vi "test_easy_linear_interpl.vi"() -> ()   [LabVIEW 2009]
doc: "Copyright (C) 2009, Stepan A. Baranov\nweb: http://www.OCTLab.org/\nemail: stepan@baranov.su"
uses:
  OCTLib.dll
panel:
  out "RSM_STAT final 2D array":dbl[](array[numeric])
  out "error out":errorcluster
  out "data Graph":dynamicdata(graph)
  out "wavelengths Graph":dynamicdata(graph)
  out "LabView final 2D array":dbl[](array[numeric])
  out "initial 2D array":dbl[](array[numeric])
  in  "stop":bool
  in  "index (row)":i32=1
  in  "Y":i32=9
  in  "X":i32=800
  in  "End wavelength":dbl=890.0
  in  "Start wavelength":dbl=800.0
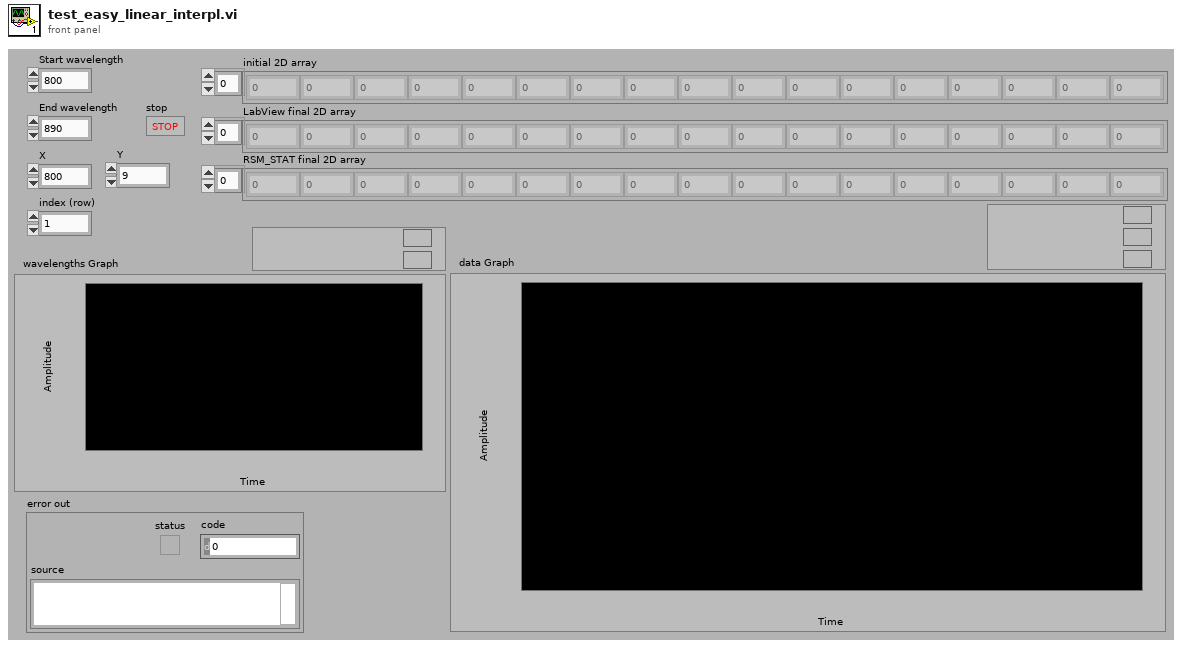
[diagram p1: front panel]
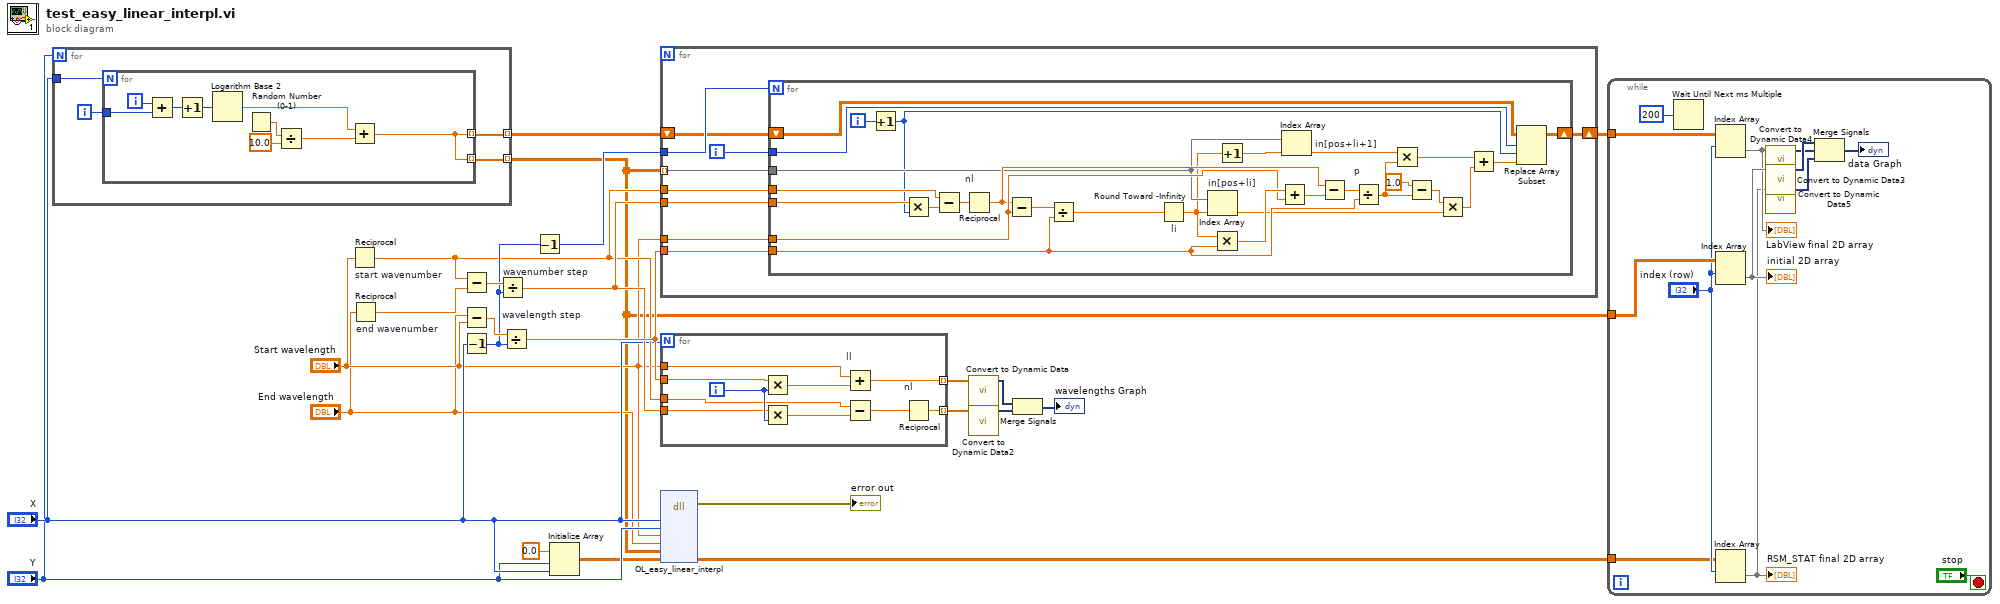
[diagram p0: block diagram]
diagram:
  n1 = for {
    N: "Y" -> [_]
    tunnel: [w28] -> w3 mode=indexing
    tunnel: "X" -> [w27]
    tunnel: [w26] -> w19 mode=indexing
    i -> [w25]
    n2 = for {
      N: w27 -> [_]
      tunnel: [w36] -> w28 mode=indexing
      tunnel: [w36] -> w26 mode=indexing
      tunnel: w25 -> [w37]
      i -> [w35]
      n3 = Add(x=w35, y=w37) -> (x+y=w34:i32)
      n4 = Increment(x=w34) -> (x+1=w33:i32)
      n5 = Logarithm Base 2(1:w33) -> (0:w32:dbl)
      n6 = Random Number (0-1)() -> (number: 0 to 1=w31:dbl)
      n7 = Divide(x=w31, y=10.0) -> (x/y=w29:dbl)
      n8 = Add(x=w32, y=w29) -> (x+y=w36:dbl)
    }
  }
  n9 = Reciprocal "start wavenumber"(x="Start wavelength") -> (1/x=w12:dbl)
  n10 = Reciprocal "end wavenumber"(x="End wavelength") -> (1/x=w23:dbl)
  n11 = Subtract(x=w12, y=w23) -> (x-y=w22:dbl)
  n12 = Subtract(x="End wavelength", y="Start wavelength") -> (x-y=w24:dbl)
  n13 = Decrement(x="X") -> (x-1=w21:i32)
  n14 = Divide "wavenumber step"(x=w22, y=w21) -> (x/y=w13:dbl)
  n15 = Divide "wavelength step"(x=w24, y=w21) -> (x/y=w17:dbl)
  n16 = Decrement(x=w21) -> (x-1=w20:i32)
  n17 = Initialize Array(0.0 ("element"), "Y", "X") -> (w2:dbl[][])
  n18 = for {
    tunnel: w20 -> [w46]
    tunnel: w3 -> [w45] mode=indexing
    tunnel: w13 -> [w44]
    tunnel: w12 -> [w43]
    tunnel: "Start wavelength" -> [w42]
    tunnel: w17 -> [w41]
    shift-right: [w39] -> w18
    shift-left: w19 -> [w40]
    i -> [w38]
    n19 = for {
      N: w46 -> [_]
      tunnel: w45 -> [w61]
      tunnel: w44 -> [w73]
      tunnel: w43 -> [w72]
      tunnel: w42 -> [w66]
      tunnel: w41 -> [w62]
      shift-right: [w47] -> w39
      shift-left: w40 -> [w51]
      tunnel: w38 -> [w50]
      i -> [w74]
      n20 = Increment(x=w74) -> (x+1=w49:i32)
      n21 = Multiply(x=w73, y=w49) -> (x*y=w71:dbl)
      n22 = Subtract(x=w72, y=w71) -> (x-y=w70:dbl)
      n23 = Reciprocal "nl"(x=w70) -> (1/x=w64:dbl)
      n24 = Subtract(x=w64, y=w66) -> (x-y=w69:dbl)
      n25 = Divide(x=w69, y=w62) -> (x/y=w68:dbl)
      n26 = Round Toward -Infinity "li"(1:w68) -> (0:w60:dbl)
      n27 = Index Array "in[pos+li]"(array=w61, index=w60) -> (element=w54:dbl)
      n28 = Multiply(x=w60, y=w62) -> (x*y=w67:dbl)
      n29 = Increment(x=w60) -> (x+1=w59:dbl)
      n30 = Add(x=w67, y=w66) -> (x+y=w65:dbl)
      n31 = Index Array "in[pos+li+1]"(array=w61, index=w59) -> (element=w58:dbl)
      n32 = Subtract(x=w64, y=w65) -> (x-y=w63:dbl)
      n33 = Divide "p"(x=w63, y=w62) -> (x/y=w57:dbl)
      n34 = Multiply(x=w58, y=w57) -> (x*y=w52:dbl)
      n35 = Subtract(x=1.0, y=w57) -> (x-y=w55:dbl)
      n36 = Multiply(x=w55, y=w54) -> (x*y=w53:dbl)
      n37 = Add(x=w52, y=w53) -> (x+y=w48:dbl)
      n38 = Replace Array Subset(array=w51, new element=w48, index (row)=w50, index (col)=w49) -> (w47:dbl[][])
    }
  }
  n39 = for {
    N: "X" -> [_]
    tunnel: w17 -> [w84]
    tunnel: "Start wavelength" -> [w82]
    tunnel: [w81] -> w16 mode=indexing
    tunnel: w13 -> [w79]
    tunnel: w12 -> [w76]
    tunnel: [w75] -> w11 mode=indexing
    i -> [w80]
    n40 = Multiply(x=w84, y=w80) -> (x*y=w83:dbl)
    n41 = Multiply(x=w79, y=w80) -> (x*y=w77:dbl)
    n42 = Add "ll"(x=w82, y=w83) -> (x+y=w81:dbl)
    n43 = Subtract(x=w76, y=w77) -> (x-y=w78:dbl)
    n44 = Reciprocal "nl"(x=w78) -> (1/x=w75:dbl)
  }
  n45 = dll-call lib="OCTLib.dll" fn="OL_easy_linear_interpl"("width"="X", "height"="Y", "start_wavelength"="Start wavelength", "end_wavelength"="End wavelength", "in"=w3, "out"=w2) -> (error out=→"error out":errorcluster, "out"=w1:dbl[][])  [unwired: 9 in, 1 out]
  n46 = call "Convert to Dynamic Data"("Array"=w16) -> ("Dynamic Data Type"=w15:dynamicdata)  [unwired: 3 in]
  n47 = call "Convert to Dynamic Data2"("Array"=w11) -> ("Dynamic Data Type"=w10:dynamicdata)  [unwired: 3 in]
  n48 = Merge Signals(w15, w10) -> (→"wavelengths Graph":dynamicdata)
  n49 = while {
    tunnel: w18 -> [w97]
    tunnel: w3 -> [w94]
    tunnel: w1 -> [w87]
    stop <- "stop" stop-if-true
    n50 = Wait Until Next ms Multiple(millisecond multiple=u32 200) -> ()  [unwired: 1 out]
    n51 = Index Array(array=w97, index (row)="index (row)") -> (element=w91:dbl[])  [unwired: 1 in]
    "LabView final 2D array" <- w91
    n52 = Index Array(array=w94, index (row)="index (row)") -> (element=w93:dbl[])  [unwired: 1 in]
    "initial 2D array" <- w93
    n53 = Index Array(array=w87, index (row)="index (row)") -> (element=w86:dbl[])  [unwired: 1 in]
    "RSM_STAT final 2D array" <- w86
    n54 = call "Convert to Dynamic Data4"("Array"=w91) -> ("Dynamic Data Type"=w90:dynamicdata)  [unwired: 3 in]
    n55 = call "Convert to Dynamic Data3"("Array"=w93) -> ("Dynamic Data Type"=w92:dynamicdata)  [unwired: 3 in]
    n56 = call "Convert to Dynamic Data5"("Array"=w86) -> ("Dynamic Data Type"=w85:dynamicdata)  [unwired: 3 in]
    n57 = Merge Signals(w92, w90, w85) -> (→"data Graph":dynamicdata)
  }
